vi "Destroy.vi"(8 "error in (no error)":errorcluster, 11 "SignalGeneratorService in":refnum<class "ServiceManagementService.lvclass">) -> (0 "error out":errorcluster, 3 "SignalGeneratorService out":refnum<class "ServiceManagementService.lvclass">)   [LabVIEW 2020, in "LineRegulation.lvlib" / "ServiceManagementService.lvclass"]
uses:
  ServiceManagementService.lvclass
  ServiceManagementService.lvclass/ServiceManagementService.ctl
  <vilib>/gRPC/LabVIEW gRPC Servicer/ServiceBase/ServiceBase.lvclass
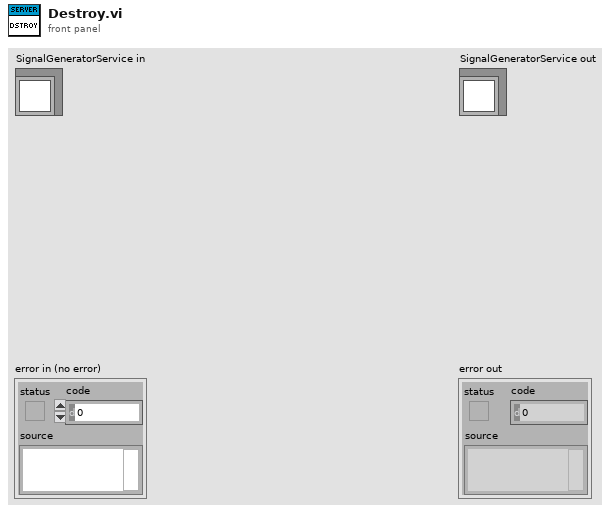
[diagram p1: front panel]
types:
  T1 = typedef "LineRegulation.lvlib/ServiceManagementService.lvclass/Server gRPC UEs.ctl" = cluster{"ni_servicemanagement_v1_ServiceManagementService_StopService gRPC UE":refnum<user-event>, "ni_measurements_servicemanagement_v1_ServiceManagementService_StopService gRPC UE":refnum<user-event>}
  T2 = typedef "LineRegulation.lvlib/ServiceManagementService.lvclass/Server Internal UEs.ctl" = cluster{"ni_servicemanagement_v1_ServiceManagementService_StopService Internal UE":refnum<user-event>, "ni_measurements_servicemanagement_v1_ServiceManagementService_StopService Internal UE":refnum<user-event>}
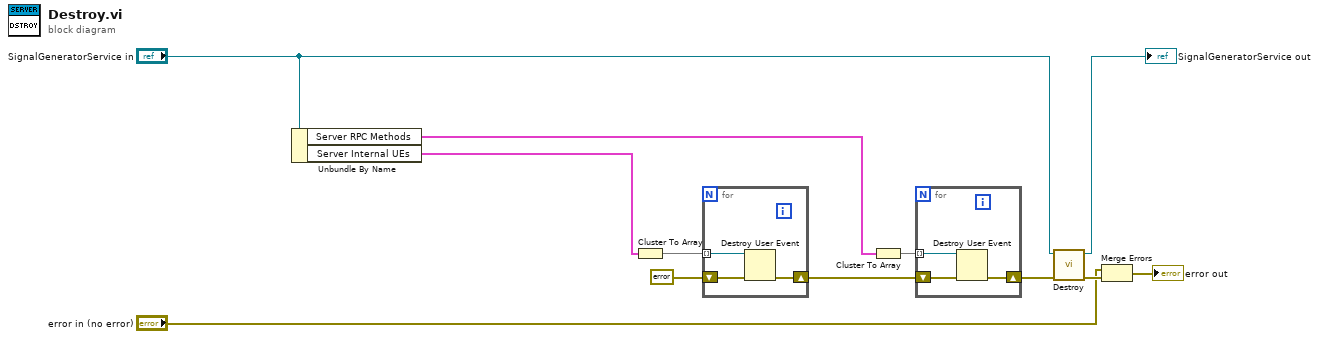
[diagram p0: block diagram]
diagram:
  n1 = Unbundle By Name("SignalGeneratorService in") -> ("Server RPC Methods"=w7:T1, "Server Internal UEs"=w8:T2)
  n2 = Cluster To Array(cluster=w8) -> (array=w9:refnum<user-event>[])
  n3 = for {
    tunnel: w9 -> [w15] mode=indexing
    shift-right: [w13] -> w5
    shift-left: errorcluster {"status"=FALSE, "code"=0, "source"=""} ("error out") -> [w14]
    n4 = Destroy User Event(user event=w15, error in=w14) -> (error out=w13:errorcluster)
  }
  n5 = Cluster To Array(cluster=w7) -> (array=w6:refnum<user-event>[])
  n6 = for {
    tunnel: w6 -> [w18] mode=indexing
    shift-right: [w16] -> w4
    shift-left: w5 -> [w17]
    n7 = Destroy User Event(user event=w18, error in=w17) -> (error out=w16:errorcluster)
  }
  n8 = call-parent "Destroy.vi"("error in (no error)"=w4, "SignalGeneratorService in"="SignalGeneratorService in") -> ("error out"=w12:errorcluster, "SignalGeneratorService out"=→"SignalGeneratorService out":refnum<class "ServiceManagementService.lvclass">)  [unwired: 8 in]
  n9 = Merge Errors("error in (no error)", w12) -> (→"error out":errorcluster)
